vi "GEOM_SortByCoords.vi"(10 "amplifiers":T1[](array[typedef]) {"fliped" items=["none", "horizontal", "vertical"]; "type" items=["LL", "LR", "UL", "UR"]}, 11 "how":enum16{"rows (y)", "columns (x)"}(ring)) -> (1 "levels":cluster{"amplifiers":i32, "coord":i32}[](array[cluster]), 2 "sorted amplifiers":T1[](array[typedef]) {"fliped" items=["none", "horizontal", "vertical"]; "type" items=["LL", "LR", "UL", "UR"]})   [LabVIEW 2016]
uses:
  GEOM_Amplifier.ctl
  GEOM_AmpType.ctl
  GEOM_ROI.ctl
  GEOM_Coords.ctl
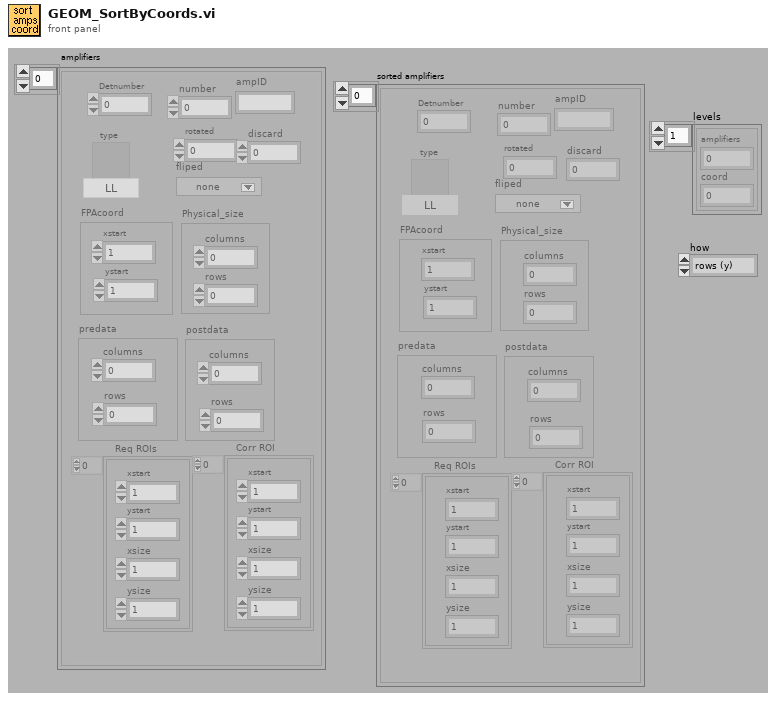
[diagram p1: front panel]
types:
  T1 = typedef "GEOM_Amplifier.ctl" = cluster{"number":i32, "type":T2, "rotated":i16, "fliped":u16, "FPAcoord":cluster{"xstart":i32, "ystart":i32}, "Physical_size":cluster{"columns":i32, "rows":i32}, "predata":cluster{"columns":i32, "rows":i32}, "postdata":cluster{"columns":i32, "rows":i32}, "Req ROIs":T3, "Corr ROI":T3, "Detnumber":i32, "ampID":string, "discard":i32}
  T2 = typedef "GEOM_AmpType.ctl" = u16
  T3 = typedef "GEOM_ROI.ctl" = T4[]
  T4 = typedef "GEOM_Coords.ctl" = cluster{"xstart":u32, "ystart":u32, "xsize":u32, "ysize":u32}
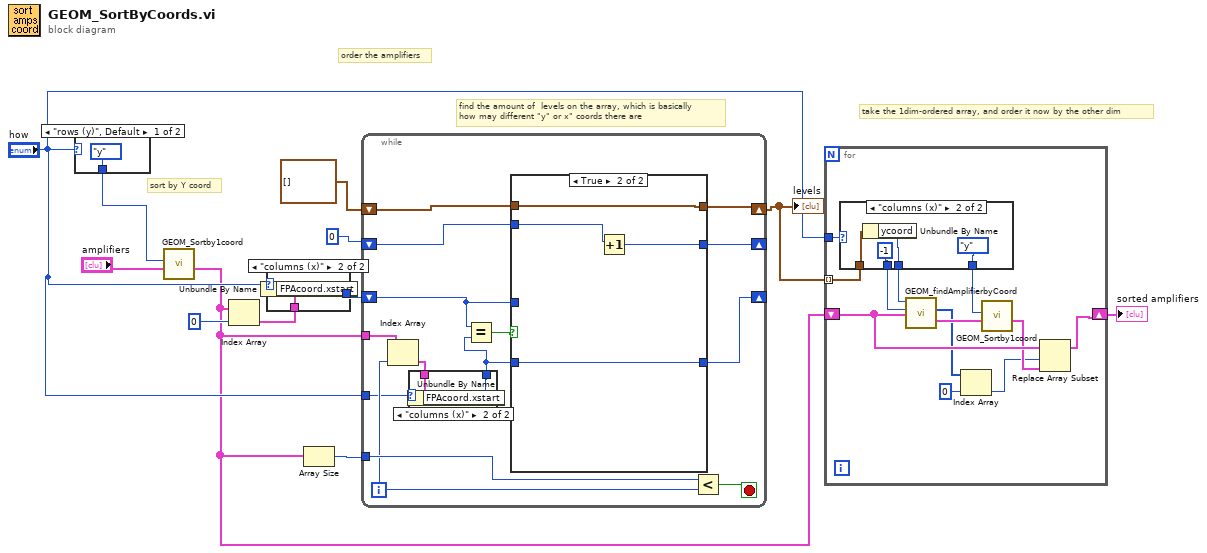
[diagram p0: block diagram]
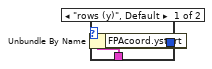
[diagram p2: hidden frame]
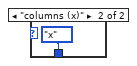
[diagram p3: hidden frame]
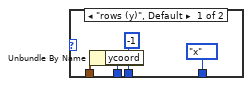
[diagram p4: hidden frame]
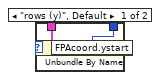
[diagram p5: hidden frame]
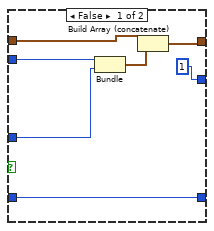
[diagram p6: hidden frame]
diagram:
  # "take the 1dim-ordered array, and order it now by the other dim"
  # "find the amount of  levels on the array, which is basically \nhow may different \"y\" or x\" coords there are"
  # "sort by Y coord"
  # "order the amplifiers"
  n1 = case shown="\"rows (y)\", Default" "how" {
    tunnel: [enum16{"x", "y"}."y" ("sort by") enum16{"x", "y"}."x" ("sort by")] -> w4
    frame "rows (y)", Default {
    }
    frame "columns (x)" {
    }
  }
  n2 = call "GEOM_Sortby1coord.vi"("amplifiers"="amplifiers", "sort by"=w4) -> ("sorted amplifiers"=w1:T1[])  [unwired: 9 out]
  n3 = Index Array(array=w1, index=0) -> (element=w8:T1)
  n4 = case shown="\"columns (x)\"" "how" {
    tunnel: w8 -> [w16 w18]
    tunnel: [w15 w17] -> w7
    frame "rows (y)", Default {
      n5 = Unbundle By Name(w16) -> ("FPAcoord.ystart"=w15:i32)
    }
    frame "columns (x)" {
      n6 = Unbundle By Name(w18) -> ("FPAcoord.xstart"=w17:i32)
    }
  }
  n7 = Array Size(array=w1) -> (size(s)=w10:i32)
  n8 = while {
    tunnel: w1 -> [w32]
    shift-right: [w28] -> _
    shift-left: w7 -> [w25]
    shift-right: [w26] -> _
    shift-left: 0 -> [w27]
    shift-right: [w24] -> w6
    shift-left: cluster{i32, "ycoord":i32}[] [] -> [w23]
    tunnel: w10 -> [w22]
    tunnel: "how" -> [w19]
    i -> [w21]
    stop <- w20 stop-if-true
    n9 = Index Array(array=w32, index=w21) -> (element=w31:T1)
    n10 = case shown="\"columns (x)\"" w19 {
      tunnel: w31 -> [w34 w36]
      tunnel: [w33 w35] -> w30
      frame "rows (y)", Default {
        n11 = Unbundle By Name(w34) -> ("FPAcoord.ystart"=w33:i32)
      }
      frame "columns (x)" {
        n12 = Unbundle By Name(w36) -> ("FPAcoord.xstart"=w35:i32)
      }
    }
    n13 = Equal?(x=w25, y=w30) -> (x = y?=w29:bool)
    n14 = case shown="True" w29 {
      tunnel: w30 -> [w42 w47]
      tunnel: [w42 w47] -> w28
      tunnel: w27 -> [w40 w46]
      tunnel: [1 w45] -> w26
      tunnel: w25 -> [w41 _]
      tunnel: [w37 w44] -> w24
      tunnel: w23 -> [w38 w44]
      frame False {
        n15 = Bundle(w40, "xstart"=w41) -> (w39:cluster{i32, "xstart":i32})  [unwired: 1 out]
        n16 = Build Array (concatenate)(w38, w39) -> (w37:cluster{i32, "xstart":i32}[])
      }
      frame True {
        n17 = Increment(x=w46) -> (x+1=w45:i32)
      }
    }
    n18 = Less?(x=w22, y=w21) -> (x < y?=w20:bool)
  }
  "levels" <- w6
  n19 = for {
    tunnel: w6 -> [w59] mode=indexing
    shift-right: [w54] -> w5
    shift-left: w1 -> [w55]
    tunnel: "how" -> [w49]
    n20 = case shown="\"columns (x)\"" w49 {
      tunnel: w59 -> [w62 w66]
      tunnel: [w61 -1 ("ycoord")] -> w58
      tunnel: [-1 ("xcoord") w65] -> w57
      tunnel: [enum16{"x", "y"}."x" ("sort by") enum16{"x", "y"}."y" ("sort by")] -> w48
      frame "rows (y)", Default {
        n21 = Unbundle By Name(w62) -> ("ycoord"=w61:i32)
      }
      frame "columns (x)" {
        n22 = Unbundle By Name(w66) -> ("ycoord"=w65:i32)
      }
    }
    n23 = call "GEOM_findAmplifierbyCoord.vi"("amplifiers"=w55, "ycoord"=w58, "xcoord"=w57) -> ("amplifiers"=w56:T1[], "indexes"=w52:i32[])  [unwired: 7 out]
    n24 = Index Array(array=w52, index=0) -> (element=w50:i32)
    n25 = call "GEOM_Sortby1coord.vi"("amplifiers"=w56, "sort by"=w48) -> ("sorted amplifiers"=w53:T1[])  [unwired: 9 out]
    n26 = Replace Array Subset(array=w55, new element=w53, index=w50) -> (w54:T1[])
  }
  "sorted amplifiers" <- w5
